vi "Current VIs Parent Directory.vi"(4 "Relative path (.)":path=path "") -> (1 "Parent Directory (+ Relative)":path)   [LabVIEW 2012, in "Path Function.lvlib"]
doc: "Gets the path to the parent directory of the calling VI. This may be used for building a path to a config file that exists in that directory or a directory relative to it. This function will move up the file structure until it reaches and Operating System Directory. It will not return the path to a built EXE or to an LLB."
uses:
  Path Function.lvlib
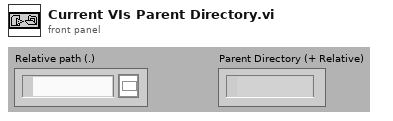
[diagram p1: front panel]
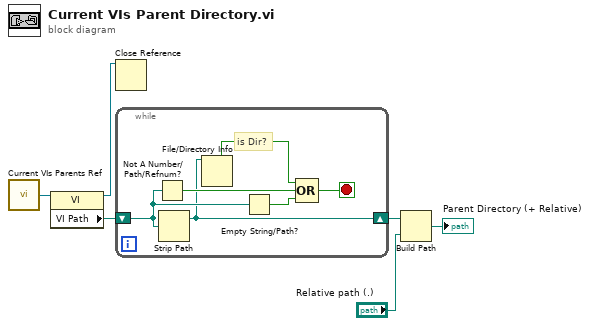
[diagram p0: block diagram]
diagram:
  n1 = call "Current VIs Parents Ref.vi"() -> ("Calling VI's Reference"=w1:refnum<vi>)  [unwired: 2 in]
  n2 = property class="VI"(reference=w1) -> (reference out=w5:refnum<vi>, "VI Path"=w6:path)  [unwired: 1 in, 1 out]
  n3 = Close Reference(reference=w5) -> ()  [unwired: 1 in, 1 out]
  n4 = while {
    shift-right: [w7] -> w2
    shift-left: w6 -> [w9]
    stop <- w11 stop-if-true
    # "is Dir?"
    n5 = Not A Number/Path/Refnum?(number/path/refnum=w9) -> (NaN/Path/Refnum?=w10:bool)
    n6 = Strip Path(path=w9) -> (stripped path=w7:path)  [unwired: 1 out]
    n7 = File/Directory Info(path=w7) -> (directory=w12:bool)  [unwired: 1 in, 6 out]
    n8 = Empty String/Path?(string/path=w9) -> (empty?=w8:bool)
    n9 = Compound Arithmetic op=OR(w12, w10, w8) -> (w11:bool)
  }
  n10 = Build Path(base path=w2, name or relative path="Relative path (.)") -> (appended path=→"Parent Directory (+ Relative)":path)
